vi "Verify new image.vi"(8 "error in (no error)":errorcluster, 11 "CCDCamera in":refnum<class "Simulated Camera.lvclass">) -> (0 "error out":errorcluster, 2 "New Images ?":bool, 3 "CCDCamera out":refnum<class "Simulated Camera.lvclass">)   [LabVIEW 2018, in "Simulated Camera.lvclass"]
doc: "Verify is there is any new image"
uses:
  Simulated Camera.lvclass
  Simulated Camera.lvclass/Simulated Camera.ctl
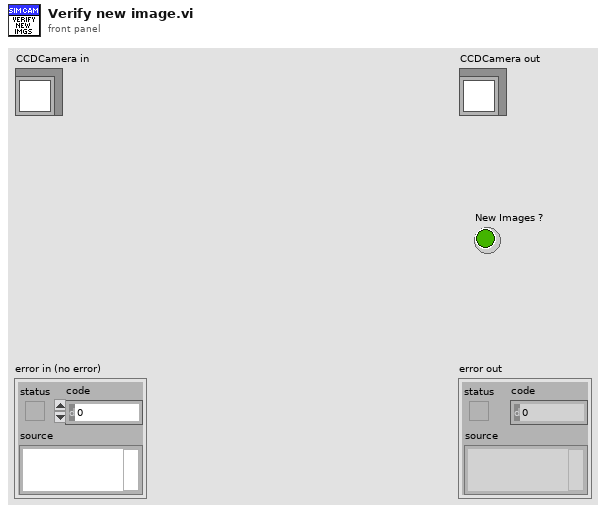
[diagram p1: front panel]
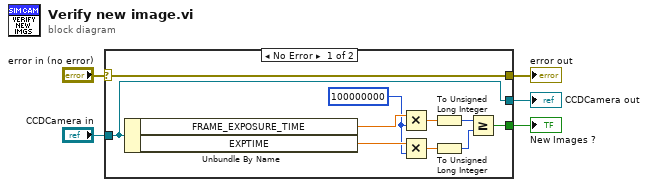
[diagram p0: block diagram]
diagram:
  n1 = case shown="No Error" "error in (no error)" {
    selector: "error in (no error)" -> [w15 w17]
    tunnel: [w15 w17] -> w4
    tunnel: [w14 w16] -> w2
    tunnel: "CCDCamera in" -> [w14 w16]
    tunnel: [w13 _] -> w1
    frame No Error {
      w10 = 100000000
      n2 = Unbundle By Name(w14) -> ("FRAME_EXPOSURE_TIME"=w12:sgl, "EXPTIME"=w11:dbl)
      n3 = Multiply(x=w12, y=w10) -> (x*y=w9:sgl)
      n4 = Multiply(x=w11, y=w10) -> (x*y=w8:dbl)
      n5 = To Unsigned Long Integer(number=w9) -> (unsigned 32bit integer=w6:u32)
      n6 = To Unsigned Long Integer(number=w8) -> (unsigned 32bit integer=w7:u32)
      n7 = Greater Or Equal?(x=w6, y=w7) -> (x >= y?=w13:bool)
    }
    frame Error {
    }
  }
  "error out" <- w4
  "CCDCamera out" <- w2
  "New Images ?" <- w1
